vi "cc_error.vi"(2 "error in (no error)":errorcluster, 3 "Error code":i32, 4 "VISA In":refnum<visa-resource-name>) -> (0 "error out":errorcluster, 1 "VISA out":refnum<visa-resource-name>)   [LabVIEW 2020]
doc: "Error Recovery"
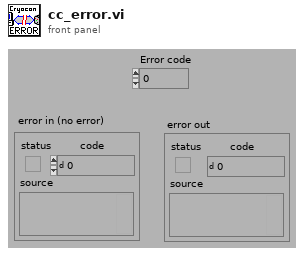
[diagram p1: front panel]
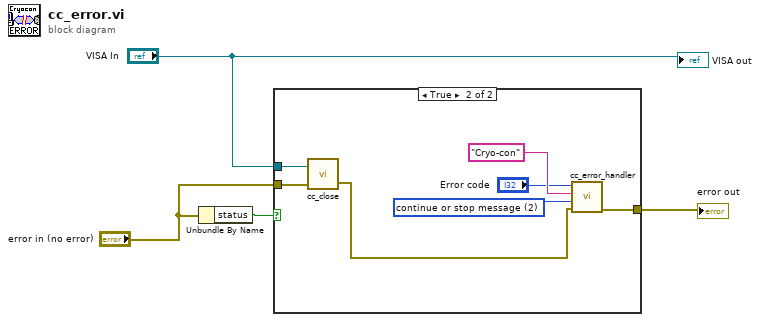
[diagram p0: block diagram]
diagram:
  n1 = Unbundle By Name("error in (no error)") -> ("status"=w4:bool)
  n2 = case shown="True" w4 {
    tunnel: "error in (no error)" -> [w5 w8]
    tunnel: [w5 w9] -> w3
    tunnel: "VISA In" -> [_ w6]
    frame False {
    }
    frame True {
      w11 = 2 items=["no dialog", "OK message", "continue or stop message"] ("type of dialog (OK msg:1)")
      n3 = call "cc_close.vi"("error in (no error)"=w8, "VISA In"=w6) -> ("error out"=w7:errorcluster)  [unwired: 1 in]
      n4 = call "cc_error_handler.vi"("error code (no error:0)"="Error code", "error source (\" \")"="Cryo-con", "type of dialog (OK msg:1)"=w11, "error in (no error)"=w7) -> ("error out"=w9:errorcluster)  [unwired: 1 in, 4 out]
    }
  }
  "error out" <- w3
  "VISA out" <- "VISA In"
